vi "Main.vi"() -> ()   [LabVIEW 2019]
uses:
  Type Def.ctl
panel:
  out "Filtered Frequency":dynamicdata(graph)
  in  "Locate Tree":bool
  out "High Winds":bool
  in  "Frequency\n in Wood in KHz":dbl min=0.0 max=1000.0 step=0.5
  out "Humidity":dbl(knob) scale=0.0..20.0
  out "CO2 Levels":dbl(knob) scale=0.0..15.0
  out "Unfiltered Acoustic\nSensor Freqency":dynamicdata(graph)
  out "Wind Speed Indicator":dbl(knob) scale=0.0..5.0
  in  "Humidity":dbl min=0.0 max=20.0 step=1.0
  in  "CO2  Levels":dbl min=0.0 max=15.0
  in  "Temperature":dbl
  in  "Wind Speed (in mph)":dbl(knob) scale=0.0..5.0
  out "on - off":bool
  in  "On / Off":bool
  out "Temperature\n    Indicator":dbl(slide) scale=0.0..100.0
  in  "Fire Alarm":bool
  in  "Temperature Warning":bool
  in  "Humidity Warning":bool
  in  "Bug Detected":bool
  in  "Force Stop":bool
  # "Pest & Fire Detector for Forest Trees"
  # "Environmental Inputs"
  # "Indicators"
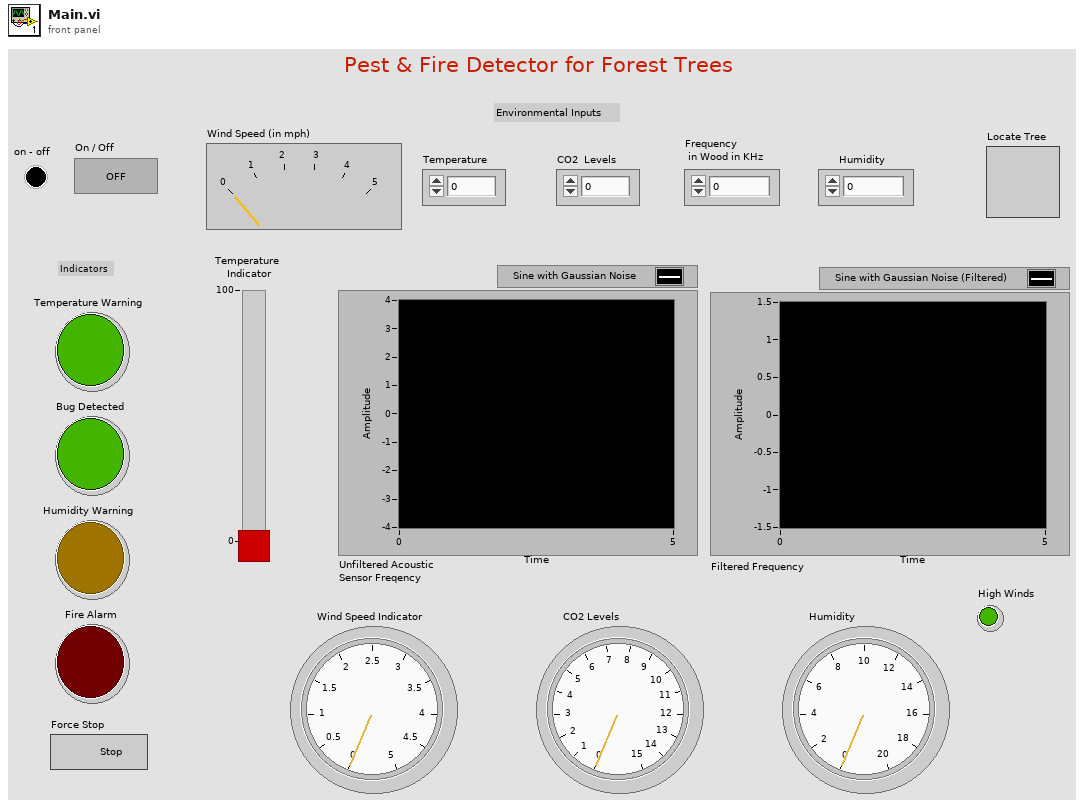
[diagram p1: front panel]
types:
  T1 = typedef "Type Def.ctl" = enum16{"Initialization", "Bug Detected", "Locate Tree", "Temp Warning", "Fire Detected", "Humidity Low", "CheckIfBug", "Idle", "Exit"}
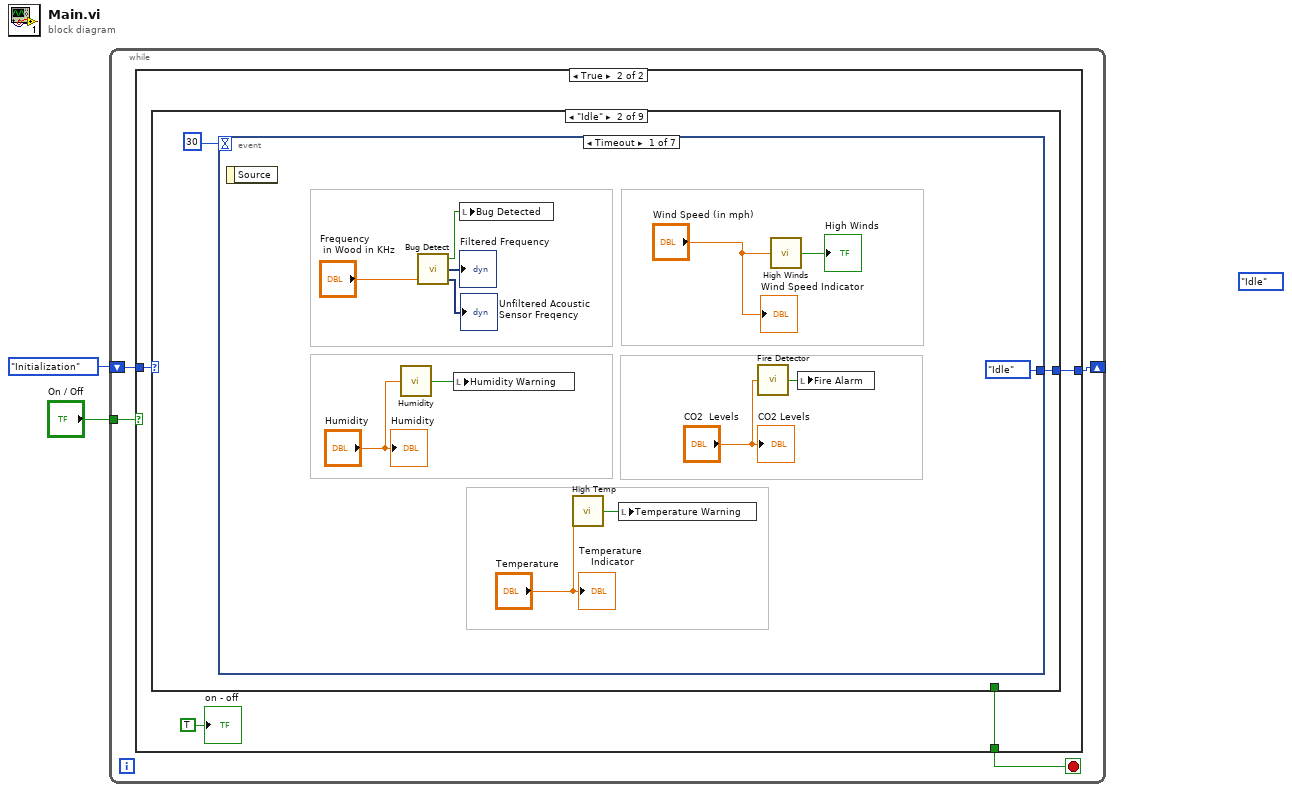
[diagram p0: block diagram]
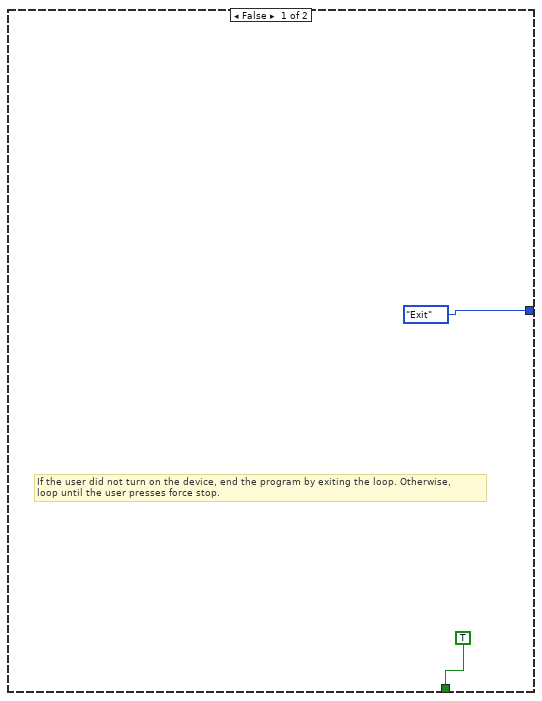
[diagram p2: hidden frame]
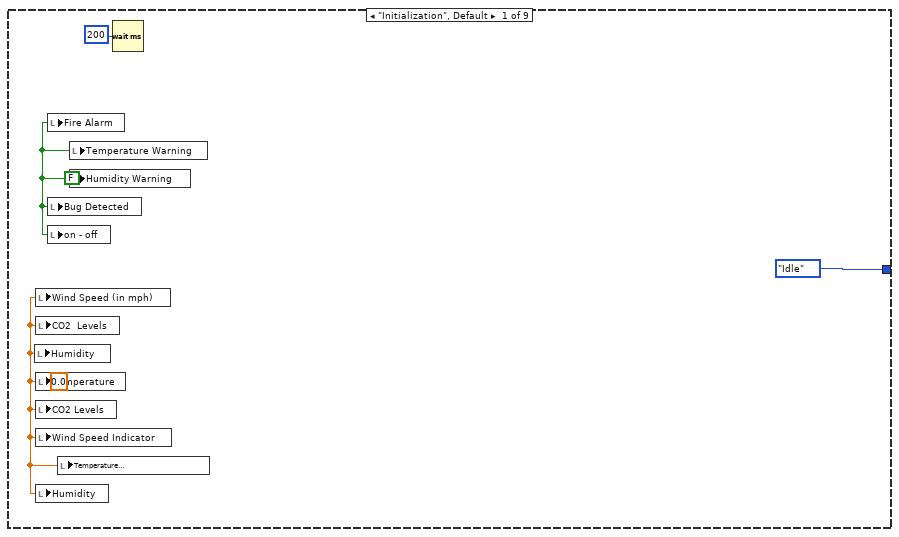
[diagram p3: hidden frame]
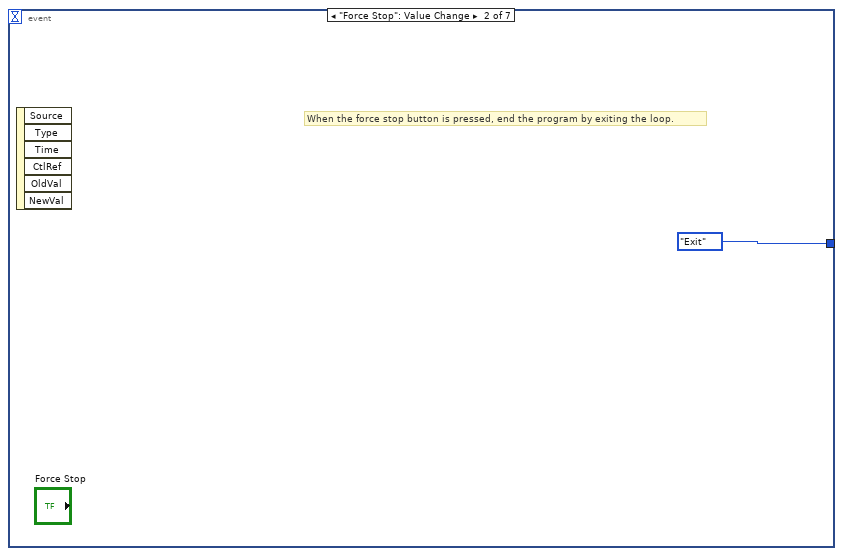
[diagram p4: hidden frame]
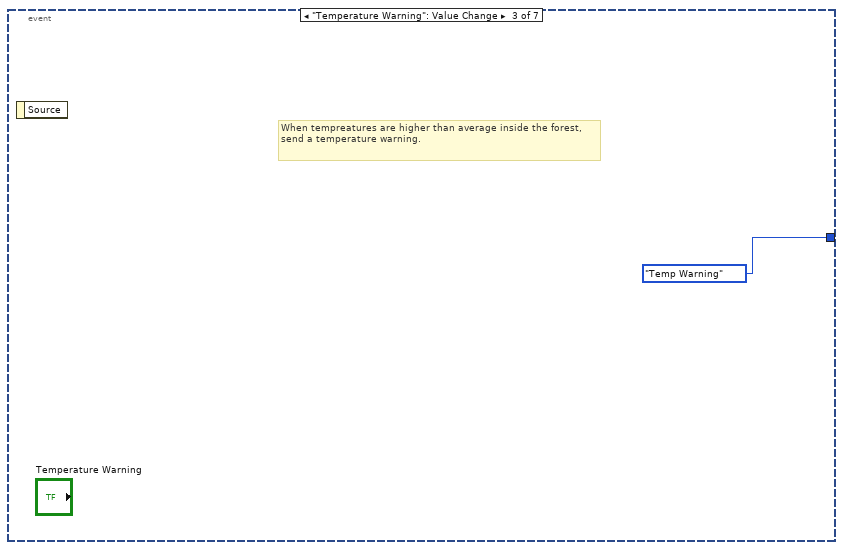
[diagram p5: hidden frame]
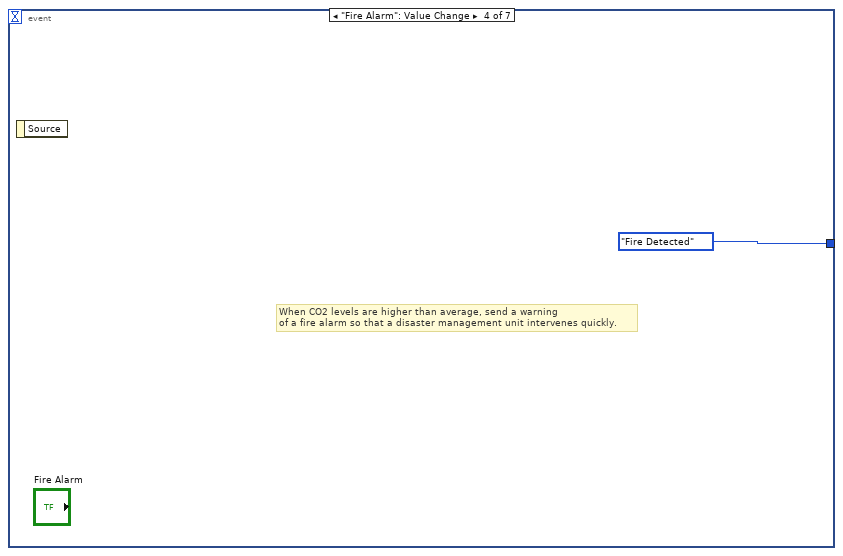
[diagram p6: hidden frame]
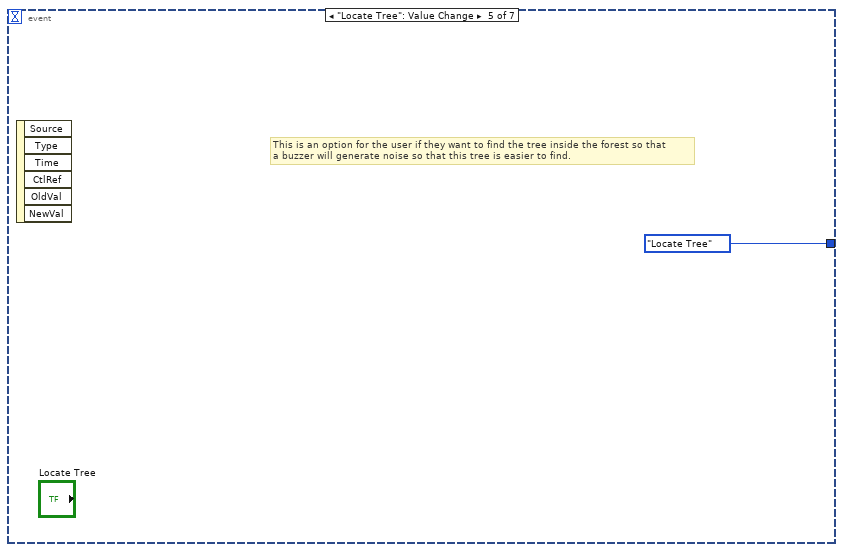
[diagram p7: hidden frame]
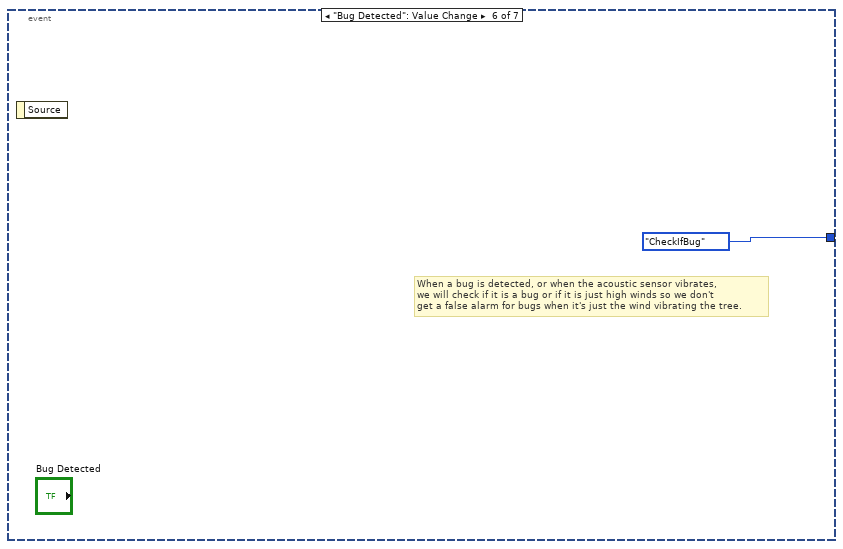
[diagram p8: hidden frame]
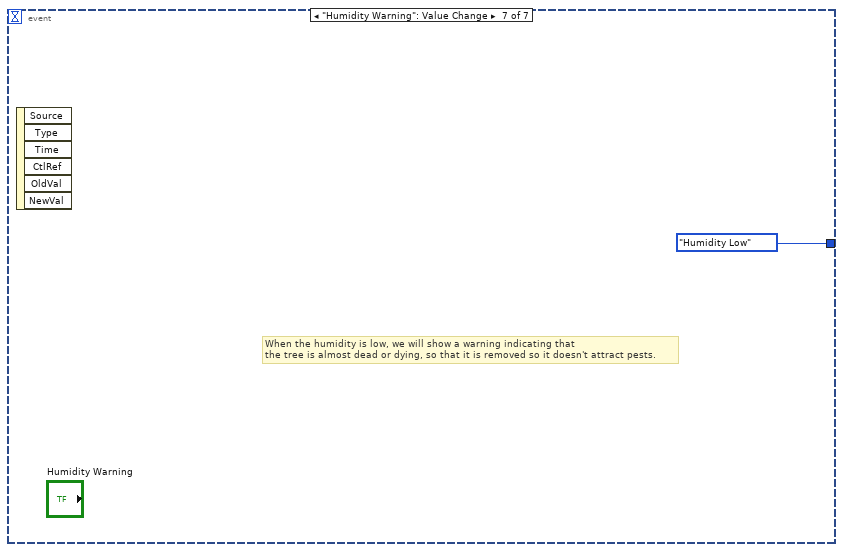
[diagram p9: hidden frame]
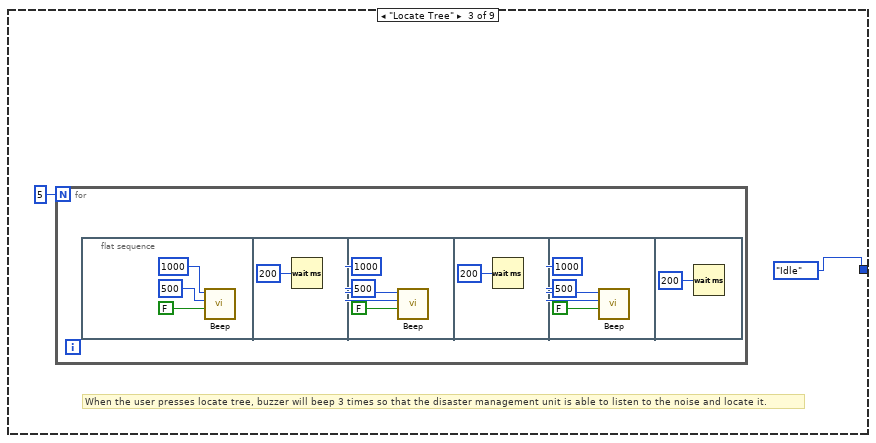
[diagram p10: hidden frame]
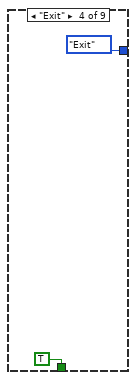
[diagram p11: hidden frame]
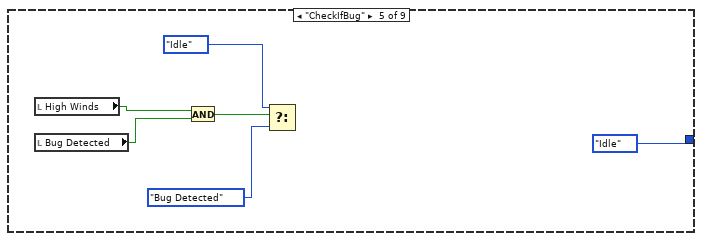
[diagram p12: hidden frame]
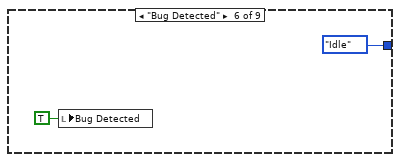
[diagram p13: hidden frame]
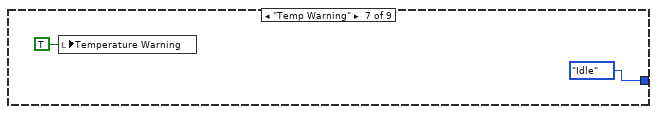
[diagram p14: hidden frame]
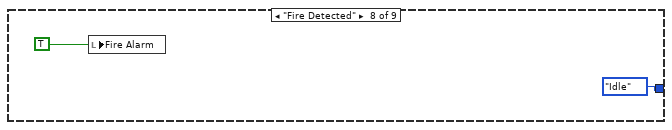
[diagram p15: hidden frame]
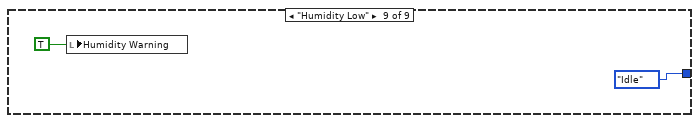
[diagram p16: hidden frame]
diagram:
  (unwired) Type_Def."Idle"
  n1 = while {
    shift-right: [w3] -> _
    shift-left: Type_Def."Initialization" -> [w4]
    tunnel: "On / Off" -> [w6]
    stop <- w5 stop-if-true
    n2 = case shown="True" w6 {
      tunnel: [TRUE w11] -> w5
      tunnel: w4 -> [_ w12]
      tunnel: [Type_Def."Exit" w9] -> w3
      frame False {
        # "If the user did not turn on the device, end the program by exiting the loop. Otherwise, \nloop until the user presses force stop."
      }
      frame True {
        n3 = case shown="\"Idle\"" w12 {
          tunnel: [_ _ _ TRUE _ _ _ _ _] -> w11
          tunnel: [Type_Def."Idle" w17 Type_Def."Idle" Type_Def."Exit" Type_Def."Idle" Type_Def."Idle" Type_Def."Idle" Type_Def."Idle" Type_Def."Idle"] -> w9
          frame "Initialization", Default {
            w16 = FALSE
            w15 = 0.0
            n4 = local write "Humidity"(w15) -> ()
            n5 = local write "Wind Speed (in mph)"(w15) -> ()
            n6 = local write "CO2  Levels"(w15) -> ()
            n7 = local write "Temperature"(w15) -> ()
            n8 = local write "CO2 Levels"(w15) -> ()
            n9 = local write "Wind Speed Indicator"(w15) -> ()
            n10 = local write "Humidity"(w15) -> ()
            n11 = local write "Fire Alarm"(w16) -> ()
            n12 = local write "Bug Detected"(w16) -> ()
            n13 = local write "on - off"(w16) -> ()
            n14 = local write "Temperature\n    Indicator"(w15) -> ()
            n15 = local write "Temperature Warning"(w16) -> ()
            n16 = local write "Humidity Warning"(w16) -> ()
            n17 = Wait (ms)(milliseconds to wait=u32 200 ("millisecond timer value")) -> ()  [unwired: 1 out]
          }
          frame "Idle" {
            n18 = event shown="[0] Timeout" {
              selector: _ -> [_ _ _ _ _ _ _]
              dyn-events: _ -> [_ _ _ _ _ _ _]
              timeout: 30 -> [_ _ _ _ _ _ _]
              tunnel: [Type_Def."Idle" Type_Def."Exit" Type_Def."Temp Warning" Type_Def."Fire Detected" Type_Def."Locate Tree" Type_Def."CheckIfBug" Type_Def."Humidity Low"] -> w17
              event Timeout {
                n19 = event-data() -> ()  [unwired: 1 in, 1 out]
                n20 = call "Humidity.vi"("Humidity"="Humidity") -> ("Humidity Warning"=w20:bool)
                n21 = call "Bug Detect.vi"("Frequency of Wood (in KHz)"="Frequency\n in Wood in KHz") -> ("Signal"=→"Unfiltered Acoustic\nSensor Freqency":dynamicdata, "Filtered signal"=→"Filtered Frequency":dynamicdata, "Bug Detected"=w22:bool)  [unwired: 2 in]
                n22 = local write "Humidity Warning"(w20) -> ()
                n23 = local write "Bug Detected"(w22) -> ()
                n24 = call "High Temp.vi"("Temperature (in *C)"="Temperature") -> ("High Temp"=w27:bool)
                n25 = local write "Temperature Warning"(w27) -> ()
                n26 = call "Fire Detector.vi"("C02 Level Input"="CO2  Levels") -> ("Boolean"=w31:bool)
                n27 = call "High Winds.vi"("Wind Speed"="Wind Speed (in mph)") -> ("High Winds"=→"High Winds":bool)
                n28 = local write "Fire Alarm"(w31) -> ()
                "CO2 Levels" <- "CO2  Levels"
                "Wind Speed Indicator" <- "Wind Speed (in mph)"
                "Temperature\n    Indicator" <- "Temperature"
                "Humidity" <- "Humidity"
              }
              event "Force Stop": Value Change {
                # "When the force stop button is pressed, end the program by exiting the loop."
                n29 = event-data() -> ()  [unwired: 1 in, 6 out]
              }
              event "Temperature Warning": Value Change {
                # "When tempreatures are higher than average inside the forest,\nsend a temperature warning."
                n30 = event-data() -> ()  [unwired: 1 in, 1 out]
              }
              event "Fire Alarm": Value Change {
                # "When CO2 levels are higher than average, send a warning\nof a fire alarm so that a disaster management unit intervenes quickly."
                n31 = event-data() -> ()  [unwired: 1 in, 1 out]
              }
              event "Locate Tree": Value Change {
                # "This is an option for the user if they want to find the tree inside the forest so that\na buzzer will generate noise so that this tree is easier to find."
                n32 = event-data() -> ()  [unwired: 1 in, 6 out]
              }
              event "Bug Detected": Value Change {
                # "When a bug is detected, or when the acoustic sensor vibrates, \nwe will check if it is a bug or if it is just high winds so we don't \nget a false alarm for bugs when it's just the wind vibrating the tree."
                n33 = event-data() -> ()  [unwired: 1 in, 1 out]
              }
              event "Humidity Warning": Value Change {
                # "When the humidity is low, we will show a warning indicating that \nthe tree is almost dead or dying, so that it is removed so it doesn't attract pests."
                n34 = event-data() -> ()  [unwired: 1 in, 6 out]
              }
            }
          }
          frame "Locate Tree" {
            # "When the user presses locate tree, buzzer will beep 3 times so that the disaster management unit is able to listen to the noise and locate it."
            n35 = for {
              N: 5 -> [_]
              n36 = flat-sequence {
                frame #0 {
                  n37 = call <vilib>:"Beep.vi"("use system alert? (T)"=FALSE, "duration (msec)"=u32 500, "frequency (Hz)"=u32 1000) -> ()  [unwired: 9 in]
                }
                frame #1 {
                  n38 = Wait (ms)(milliseconds to wait=u32 200) -> ()  [unwired: 1 out]
                }
                frame #2 {
                  n39 = call <vilib>:"Beep.vi"("use system alert? (T)"=FALSE, "duration (msec)"=u32 500, "frequency (Hz)"=u32 1000) -> ()  [unwired: 9 in]
                }
                frame #3 {
                  n40 = Wait (ms)(milliseconds to wait=u32 200) -> ()  [unwired: 1 out]
                }
                frame #4 {
                  n41 = call <vilib>:"Beep.vi"("use system alert? (T)"=FALSE, "duration (msec)"=u32 500, "frequency (Hz)"=u32 1000) -> ()  [unwired: 9 in]
                }
                frame #5 {
                  n42 = Wait (ms)(milliseconds to wait=u32 200) -> ()  [unwired: 1 out]
                }
              }
            }
          }
          frame "Exit" {
          }
          frame "CheckIfBug" {
            n43 = local read "High Winds"() -> (w59:bool)
            n44 = local read "Bug Detected"() -> (w58:bool)
            n45 = And(x=w59, y=w58) -> (x .and. y?=w57:bool)
            n46 = Select(t=Type_Def."Idle", s=w57, f=Type_Def."Bug Detected") -> ()  [unwired: 1 out]
          }
          frame "Bug Detected" {
            n47 = local write "Bug Detected"(TRUE ("Bug Detected")) -> ()
          }
          frame "Temp Warning" {
            n48 = local write "Temperature Warning"(TRUE ("Temperature Warning")) -> ()
          }
          frame "Fire Detected" {
            n49 = local write "Fire Alarm"(TRUE ("Temperature Warning")) -> ()
          }
          frame "Humidity Low" {
            n50 = local write "Humidity Warning"(TRUE ("Temperature Warning")) -> ()
          }
        }
        "on - off" <- TRUE ("on - off")
      }
    }
  }
